vi "LinVer Protokoll_Auswertung.vi"(0 "Sollwerte":sgl[](array[numeric]), 1 "Bedingung:":T1, 5 "Istwerte":sgl[](array[numeric]), 7 "Konzentration":sgl, 9 "Maximale Abweichung":sgl, 11 "error in (no error)":errorcluster caption="Fehler (Eingang, kein Fehler)") -> (4 "Auswertung":string[](array[string]), 6 "Auswertung":cluster{sgl[], sgl[], bool[]}, 15 "error out":errorcluster caption="Fehler (Ausgang)")   [LabVIEW 2020, in "Linearisierung v2.lvlib" / "Linearity verification 1065-307.lvlib"]
uses:
  Linearity verification 1065-307.lvlib
  Bedingung.ctl
  <vilib>/Analysis/6fits.llb/Curve Fitting Criteria.ctl
  Aktion FGV Auswertung sammeln.ctl
  Sprachverwaltung/FGV Aktion Tabelle zerlegen.ctl
  <vilib>/Analysis/NI_AALPro.lvlib
  Sprachverwaltung/Sprachverwaltung.lvlib
  Allgemein/allgemeine Sub-VIs.lvlib
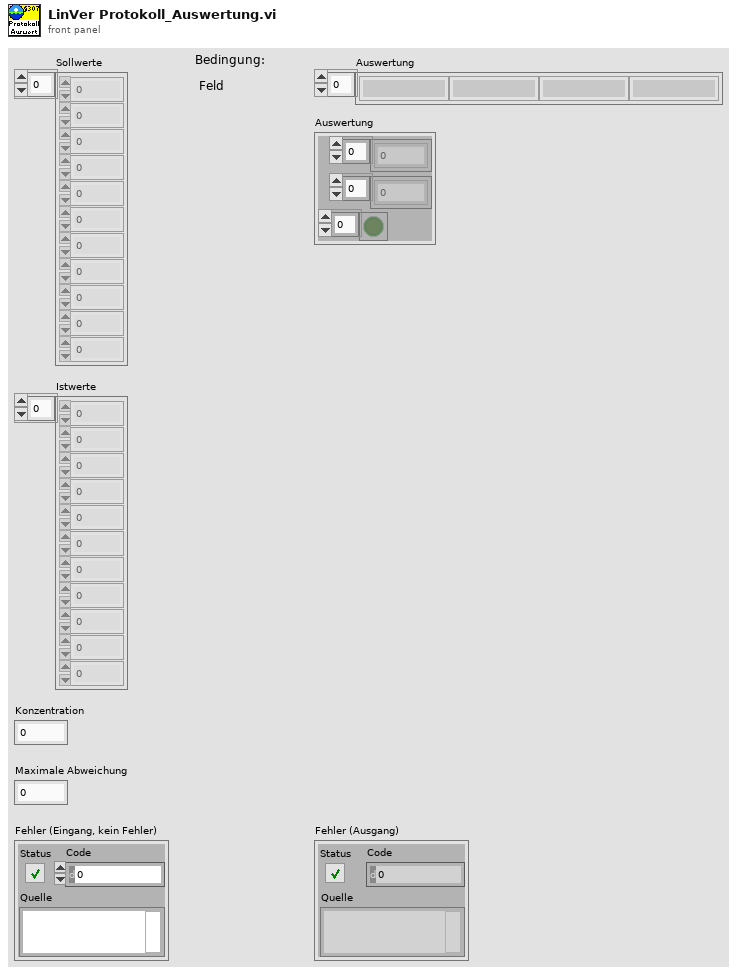
[diagram p1: front panel]
types:
  T1 = typedef "Linearisierung v2.lvlib/Linearity verification 1065-307.lvlib/Bedingung.ctl" = enum16{"Feld", "Labor"}
  T2 = typedef "Sprachverwaltung.lvlib/FGV Aktion Tabelle zerlegen.ctl" = enum16{"laden", "vereinzeln", "speichern"}
  T3 = typedef "Linearisierung v2.lvlib/Linearity verification 1065-307.lvlib/Aktion FGV Auswertung sammeln.ctl" = enum16{"lesen", "Auswertung", "löschen"}
  T4 = typedef "NI_AALPro.lvlib/Curve Fitting Criteria.ctl" = u16
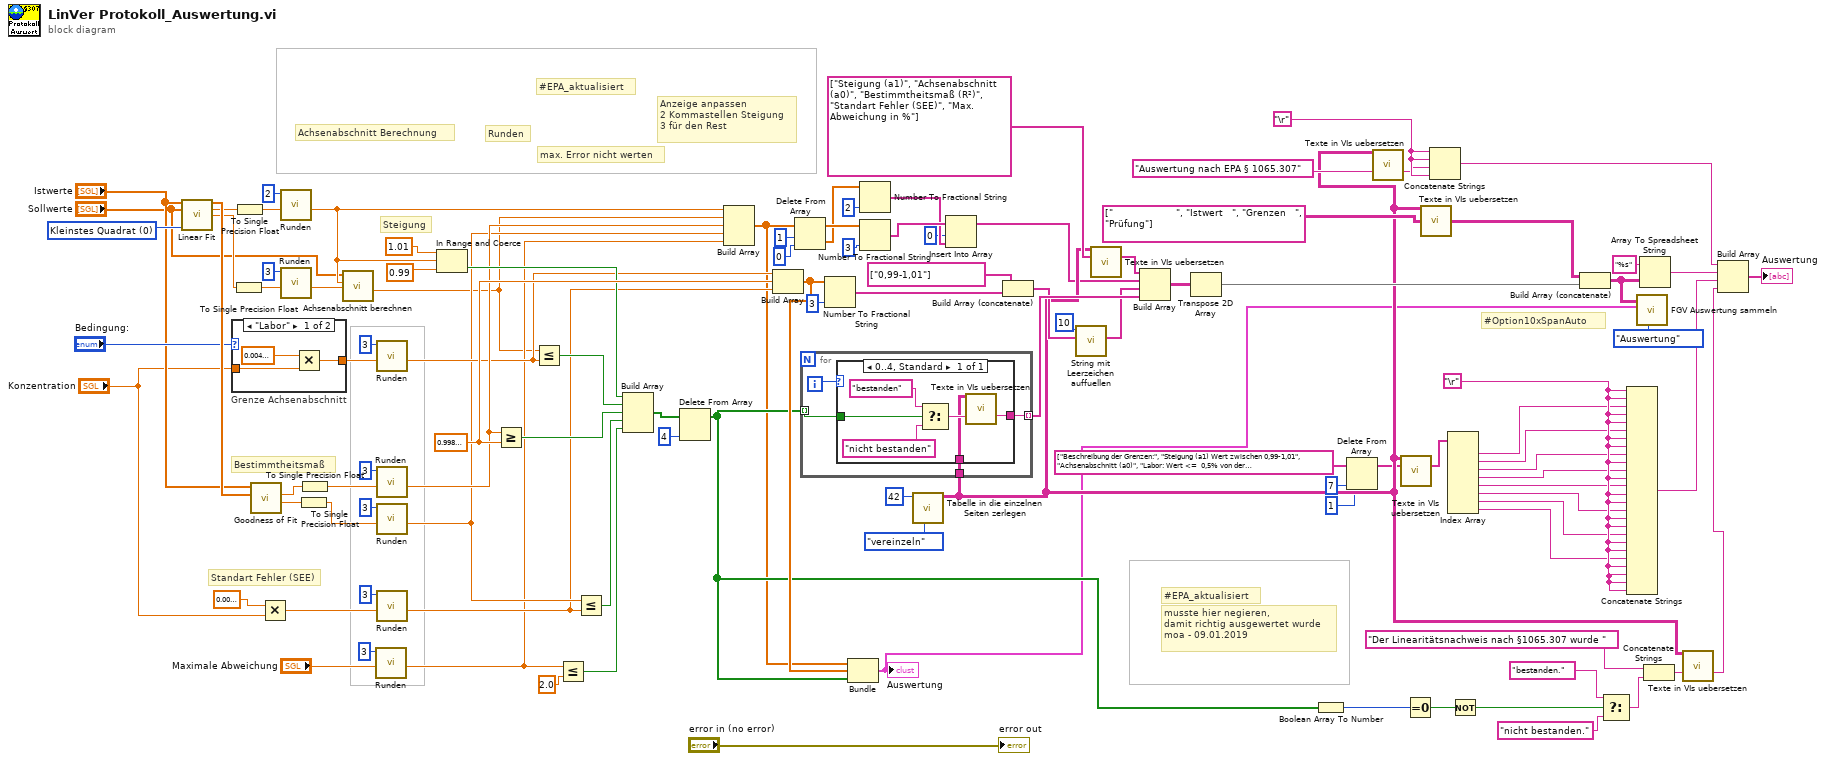
[diagram p0: block diagram]
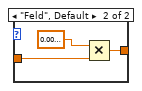
[diagram p2: hidden frame]
diagram:
  w65 = "\r"
  w67 = "\r"
  w90 = sgl 0.998 ("x")
  w103 = T4 0 items=["Kleinstes Quadrat", "Kleinstes absolutes Residuum", "Biquadrat"] ("method")
  # "#Option10xSpanAuto"
  # "max. Error nicht werten"
  # "musste hier negieren,\ndamit richtig ausgewertet wurde\nmoa - 09.01.2019"
  # "#EPA_aktualisiert"
  # "Achsenabschnitt Berechnung"
  # "Runden"
  # "Anzeige anpassen\n2 Kommastellen Steigung\n3 für den Rest"
  # "#EPA_aktualisiert"
  # "Bestimmtheitsmaß"
  # "Steigung"
  # "Standart Fehler (SEE)"
  n1 = call <vilib>:"Linear Fit.vi"("Y"="Istwerte", "X"="Sollwerte", "method"=w103) -> ("Best Linear Fit"=w108:dbl[], "slope"=w102:dbl, "intercept"=w101:dbl)  [unwired: 8 in, 2 out]
  n2 = case "Grenze Achsenabschnitt" shown="\"Labor\"" "Bedingung:" {
    tunnel: "Konzentration" -> [w111 w114]
    tunnel: [w109 w112] -> w29
    frame "Labor" {
      n3 = Multiply(x=sgl 0.005, y=w111) -> (x*y=w109:sgl)
    }
    frame "Feld", Default {
      n4 = Multiply(x=sgl 0.01, y=w114) -> (x*y=w112:sgl)
    }
  }
  n5 = To Single Precision Float(number=w101) -> (single precision float=w31:sgl)
  n6 = To Single Precision Float(number=w102) -> (single precision float=w43:sgl)
  n7 = call <vilib>:"Goodness of Fit.vi"("Best Fit"=w108, "Y"="Istwerte") -> ("RMSE"=w99:dbl, "R-square"=w100:dbl)  [unwired: 6 in, 2 out]
  n8 = Multiply(x=sgl 0.01, y="Konzentration") -> (x*y=w23:sgl)
  n9 = call "Runden.vi"("Wert"=w43, "Stellen"=2) -> ("gerundeter Wert"=w6:dbl)  [unwired: 8 in, 1 out]
  n10 = call "Runden.vi"("Wert"=w31, "Stellen"=3) -> ("gerundeter Wert"=w7:dbl)  [unwired: 8 in, 1 out]
  n11 = To Single Precision Float(number=w99) -> (single precision float=w26:sgl)
  n12 = To Single Precision Float(number=w100) -> (single precision float=w42:sgl)
  n13 = call "Achsenabschnitt berechnen.vi"("Achsenabschnitt"=w7, "Steigung"=w6, "xmin"="Sollwerte") -> ("Intercept"=w5:dbl)  [unwired: 8 in]
  n14 = call "Runden.vi"("Wert"="Maximale Abweichung", "Stellen"=3) -> ("gerundeter Wert"=w19:dbl)  [unwired: 8 in, 1 out]
  n15 = call "Runden.vi"("Wert"=w29, "Stellen"=3) -> ("gerundeter Wert"=w28:dbl)  [unwired: 8 in, 1 out]
  n16 = call "Runden.vi"("Wert"=w42, "Stellen"=3) -> ("gerundeter Wert"=w40:dbl)  [unwired: 8 in, 1 out]
  n17 = call "Runden.vi"("Wert"=w26, "Stellen"=3) -> ("gerundeter Wert"=w25:dbl)  [unwired: 8 in, 1 out]
  n18 = call "Runden.vi"("Wert"=w23, "Stellen"=3) -> ("gerundeter Wert"=w22:dbl)  [unwired: 8 in, 1 out]
  n19 = In Range and Coerce(upper limit=1.01 ("Obergrenze"), x=w6, lower limit=0.99 ("Untergrenze")) -> (In Range?=w89:bool)  [unwired: 1 out]
  n20 = Greater Or Equal?(x=w40, y=w90) -> (x >= y?=w87:bool)
  n21 = Less Or Equal?(x=w5, y=w28) -> (x <= y?=w88:bool)
  n22 = Less Or Equal?(x=w19, y=sgl 2.0 ("Element")) -> (x <= y?=w75:bool)
  n23 = Less Or Equal?(x=w25, y=w22) -> (x <= y?=w86:bool)
  n24 = Build Array(w89, w88, w87, w86, w75) -> (w38:bool[])
  n25 = Delete From Array(array=w38, index=4 ("Index")) -> (array with subset deleted=w37:bool[])  [unwired: 1 in, 1 out]
  n26 = Build Array(w6, w5, w40, w25, w19) -> (w16:dbl[])
  n27 = Build Array(w28, w90, w22) -> (w79:dbl[])
  n28 = Delete From Array(array=w16, length=1 ("Länge"), index=0 ("Index")) -> (deleted portion=w12:dbl[], array with subset deleted=w14:dbl[])
  n29 = Number To Fractional String(number=w79, precision (6)=i16 3 ("Genauigkeit (6)")) -> (F-format string=w96:string[])  [unwired: 2 in]
  n30 = Bundle(w16, w79, w37) -> (w1:cluster{dbl[], dbl[], bool[]})  [unwired: 1 in]
  "Auswertung" <- w1
  n31 = Number To Fractional String(number=w12, precision (6)=i16 2 ("Genauigkeit (6)")) -> (F-format string=w10:string[])  [unwired: 2 in]
  n32 = Number To Fractional String(number=w14, precision (6)=i16 3 ("Genauigkeit (6)")) -> (F-format string=w11:string[])  [unwired: 2 in]
  n33 = call "Tabelle in die einzelnen Seiten zerlegen.vi"("Aktion"=FGV_Aktion_Tabelle_zerlegen."vereinzeln", "Index (Seite)"=42) -> ("Sprachliste"=w45:string[][])  [unwired: 7 in, 2 out]
  n34 = for {
    tunnel: w37 -> [w118] mode=indexing
    tunnel: [w117] -> w85 mode=indexing
    tunnel: w45 -> [w116]
    i -> [w115]
    n35 = case shown="0..4, Standard" w115 {
      tunnel: w118 -> [w122]
      tunnel: [w120] -> w117
      tunnel: w116 -> [w119]
      frame 0..4, Default {
        n36 = Select(t="bestanden", s=w122, f="nicht bestanden") -> (s? t:f=w121:string)
        n37 = call "Texte in VIs uebersetzen.vi"("Sprachliste"=w119, "String zum Übersetzen"=w121) -> ("String zum Übersetzen"=w120:string)  [unwired: 9 in, 4 out]
      }
    }
  }
  n38 = Insert Into Array(array=w11, index=0 ("Index"), new element=w10) -> (w17:string[])
  n39 = Build Array (concatenate)(string[] ["0,99-1,01"] ("Element"), w96) -> (w82:string[])
  n40 = call "String mit Leerzeichen auffuellen.vi"("1 Dimension"=w82, "gewünschte Stringgröße"=10) -> ("1 Dimension"=w80:string[])  [unwired: 8 in, 1 out]
  n41 = call "Texte in VIs uebersetzen.vi"("Sprachliste"=w45, "String-Array zum Übersetzen"=string[] ["Steigung (a1)", "Achsenabschnitt (a0)", "Bestimmtheitsmaß (R²)", "Standart Fehler (SEE)", "Max. Abweichung in %"]) -> ("String-Array zum Übersetzen"=w52:string[])  [unwired: 9 in, 4 out]
  n42 = Build Array(w52, w17, w80, w85) -> (w93:string[][])
  n43 = Transpose 2D Array(2D array=w93) -> (transposed array=w92:string[][])
  n44 = Boolean Array To Number(Boolean array=w37) -> (number=w72:u32)
  n45 = Delete From Array(array=string[] ["Beschreibung der Grenzen:", "Steigung (a1) Wert zwischen 0,99-1,01", "Achsenabschnitt (a0)", "Labor: Wert <=  0,5% von der Kalibriergaskonzentration", "Feld: Wert <=  1% von der Kalibriergaskonzentration", "Bestimmtheitsmaß (R²) Wert >= 0,998", "Standart Fehler (SEE) Wert <= 1% von der Kalibriergaskonzentration", "Max. Abweichung in % <= 2% von der Kalibriergaskonzentration"], length=1 ("Länge"), index=7 ("Index")) -> (array with subset deleted=w36:string[])  [unwired: 1 out]
  n46 = call "Texte in VIs uebersetzen.vi"("Sprachliste"=w45, "String zum Übersetzen"="Auswertung nach EPA § 1065.307") -> ("String zum Übersetzen"=w48:string)  [unwired: 9 in, 4 out]
  n47 = call "Texte in VIs uebersetzen.vi"("Sprachliste"=w45, "String-Array zum Übersetzen"=w36) -> ("String-Array zum Übersetzen"=w62:string[])  [unwired: 9 in, 4 out]
  n48 = Equal To 0?(x=w72) -> (x = 0?=w71:bool)
  n49 = call "Texte in VIs uebersetzen.vi"("Sprachliste"=w45, "2D String-Array zum Übersetzen"=string[][] [["                     ", "Istwert   ", "Grenzen   ", "Prüfung"]]) -> ("2D String-Array zum Übersetzen"=w46:string[][])  [unwired: 9 in, 4 out]
  n50 = Concatenate Strings(w65, w65, w48, w65) -> (w66:string)
  n51 = Index Array(array=w62) -> (element #1=w61:string, element #2=w60:string, element #3=w59:string, element #4=w58:string, element #5=w57:string, element #6=w56:string, element #7=w55:string, element #8=w54:string)  [unwired: 8 in]
  n52 = Not(x=w71) -> (.not. x?=w8:bool)
  n53 = Build Array (concatenate)(w46, w92) -> (w77:string[][])
  n54 = Select(t="bestanden.", s=w8, f="nicht bestanden.") -> (s? t:f=w69:string)
  n55 = Concatenate Strings(w67, w67, w61, w67, w67, w60, w67, w67, w59, w67, w58, w67, w57, w67, w67, w56, w67, w67, w55, w67, w67, w54, w67, w67, w67, w67) -> (w68:string)
  n56 = call "FGV Auswertung sammeln.vi"("Aktion"=Aktion_FGV_Auswertung_sammeln."Auswertung", "Auswertung"=w1, "LINVer Auswertung"=w77) -> ()  [unwired: 6 in, 3 out]
  n57 = Array To Spreadsheet String(array=w77, 3:"%s" ("Format-String")) -> (spreadsheet string=w84:string)  [unwired: 1 in]
  n58 = Concatenate Strings("Der Linearitätsnachweis nach §1065.307 wurde ", w69) -> (w51:string)
  n59 = call "Texte in VIs uebersetzen.vi"("Sprachliste"=w45, "String zum Übersetzen"=w51) -> ("String zum Übersetzen"=w50:string)  [unwired: 9 in, 4 out]
  n60 = Build Array(w66, w84, w68, w50) -> (→"Auswertung":string[])
  "error out" <- "error in (no error)"
